vi "robot set cooperation fun state.vi"(0 "robot_id":i32, 5 "enable":bool, 11 "error in (no error)":errorcluster caption="错误输入（无错误）") -> (4 "robot_id out":i32, 8 "function return":i32, 15 "error out":errorcluster caption="错误输出")   [LabVIEW 2020, in "small_scara_interface.lvlib"]
doc: "extern \"C\" __declspec(dllexport) int robot_set_cooperation_fun_state(int robot_id, bool enable);"
uses:
  <instrlib>/Robot-HL/small_scara_interface/small_scara_interface.lvlib
  <instrlib>/Robot-HL/small_scara_interface/small_scara_interface.dll
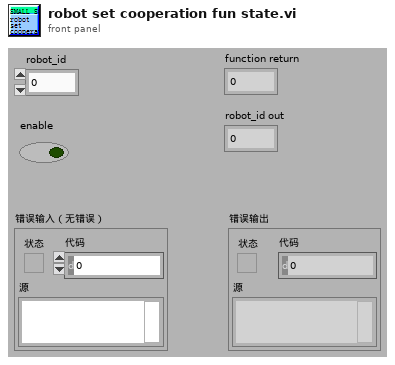
[diagram p1: front panel]
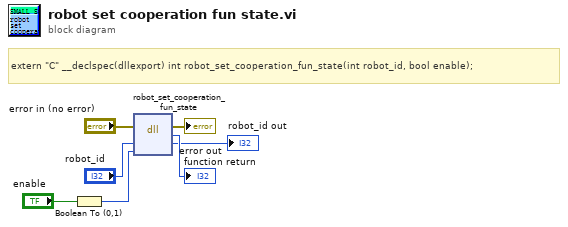
[diagram p0: block diagram]
diagram:
  # "extern \"C\" __declspec(dllexport) int robot_set_cooperation_fun_state(int robot_id, bool enable);"
  n1 = Boolean To (0,1)(Boolean="enable") -> (0, 1=w4:i16)
  n2 = dll-call lib="C:/Program Files/National Instruments/LabVIEW 2020/instr.lib/Robot-HL/small_scara_interface/small_scara_interface.*" fn="robot_set_cooperation_fun_state"(error in="error in (no error)", "robot_id"="robot_id", "enable"=w4) -> (error out=→"error out":errorcluster, "返回类型"=→"function return":i32, "robot_id"=→"robot_id out":i32)  [unwired: 3 in, 1 out]
